vi "Execute Build Target.vi"(7 "LabVIEW Previous Version":T1=enum."2015", 8 "Error In":errorcluster, 11 "Target Project Root In":path) -> (0 "Error Out":errorcluster, 3 "Target Project Root Out":path)   [LabVIEW 2017, in "Scripts.lvlib"]
doc: "Executes building a project/target using the System Exec.vi to start a specific version of LabVIEW with the \"Build Target.vi\" as an argument. Since the \"Build Target.vi\" is configured to run when loaded, this will immediate build all of the components and the VI package from within the specific version of LabVIEW.\n\nThe VI Server cannot be used here. The System Exec.vi must be used to ensure the correct version of LabVIEW is used to open and run the \"Build Target.vi\". The VI Server will use the LabVIEW environment that is executing this VI, not the correct version."
uses:
  Scripts.lvlib
  Controls/LabVIEW Versions.ctl
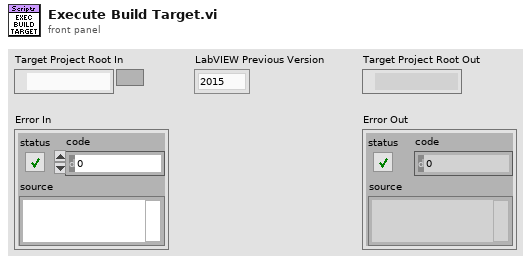
[diagram p1: front panel]
types:
  T1 = typedef "Scripts.lvlib/LabVIEW Versions.ctl" = enum16{"2009", "2010", "2011", "2012", "2013", "2014", "2015", "2016", "2017", "2018"}
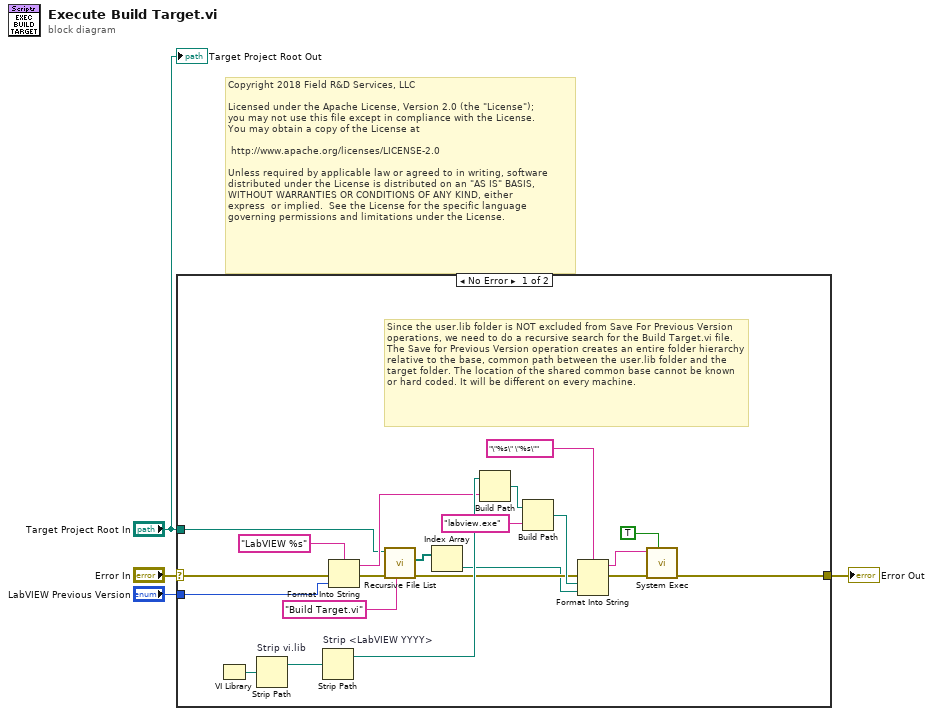
[diagram p0: block diagram]
diagram:
  # "Copyright 2018 Field R&D Services, LLC\n\nLicensed under the Apache License, Version 2.0 (the \"License\");\nyou may not use this file except in compliance with the License.\nYou may obtain a copy of the License at\n\n\thttp://www.apache.org/licenses/LICENSE-2.0\n\nUnless required by applicable law or agreed to in writing, software\ndistributed under the License is distributed on an \"AS IS\" BASIS,\nWITHOUT WARRANTIES OR CONDITIONS OF ANY KIND, either \nexpress  or implied.  See the License for the specific language \ngoverning permissions and limitations under the License."
  n1 = case shown="No Error" "Error In" {
    selector: "Error In" -> [w5 w26]
    tunnel: [w18 w26] -> w4
    tunnel: "LabVIEW Previous Version" -> [w12 _]
    tunnel: "Target Project Root In" -> [w9 _]
    frame No Error {
      # "Since the user.lib folder is NOT excluded from Save For Previous Version operations, we need to do a recursive search for the Build Target.vi file. The Save for Previous Version operation creates an entire folder hierarchy relative to the base, common path between the user.lib folder and the target folder. The location of the shared common base cannot be known or hard coded. It will be different on every machine."
      n2 = VI Library() -> (path=w25:path)
      n3 = Strip Path "Strip vi.lib"(path=w25) -> (stripped path=w24:path)  [unwired: 1 out]
      n4 = Strip Path "Strip <LabVIEW YYYY>"(path=w24) -> (stripped path=w23:path)  [unwired: 1 out]
      n5 = Format Into String(format string="LabVIEW %s", error in=w5, w12) -> (resulting string=w21:string, error out=w11:errorcluster)  [unwired: 1 in]
      n6 = call <vilib>:"Recursive File List.vi"("pattern"="Build Target.vi", "error in (no error)"=w11, "Folder Path"=w9) -> ("error out"=w10:errorcluster, "All Files in Dir"=w7:path[])  [unwired: 4 in, 3 out]
      n7 = Index Array(array=w7) -> (element=w6:path)  [unwired: 1 in]
      n8 = Build Path(base path=w23, name or relative path=w21) -> (appended path=w20:path)
      n9 = Build Path(base path=w20, name or relative path="labview.exe") -> (appended path=w15:path)
      n10 = Format Into String(format string="\"%s\" \"%s\"", error in=w10, w15, w6) -> (resulting string=w14:string, error out=w17:errorcluster)  [unwired: 1 in]
      n11 = call <vilib>:"System Exec.vi"("wait until completion? (T)"=TRUE, "error in (no error)"=w17, "command line"=w14) -> ("error out"=w18:errorcluster)  [unwired: 5 in, 3 out]
    }
    frame Error {
    }
  }
  "Error Out" <- w4
  "Target Project Root Out" <- "Target Project Root In"
